vi "DAQX mod 1SDI v02.vi"(0 "resource name":refnum<k15>="PXI1Slot2", 1 "close (T)":bool=TRUE, 2 "Record Data":bool, 3 "numSamples":i32=-1, 4 "max time (s)":dbl=10.0 caption="max time", 5 "min sample rate":dbl=100000000.0, 6 "File location":path, 7 "error in":errorcluster, 8 "reference position":dbl=50.0, 9 "Additional text":string, 10 "Type of measurement":T2, 11 "Name root":string, 13 "channel parameters":T4(array[cluster])=[{"channel name"="0", "input impedance"=0, "maximum input frequency"=30000000.0, "vertical coupling"=1, "probe attenuation"=1.0, "vertical range"=2.0, "vertical offset"=0.0, "channel enabled"=TRUE}, {"channel name"="1", "input impedance"=0, "maximum input frequency"=30000000.0, "vertical coupling"=1, "probe attenuation"=1.0, "vertical range"=2.0, "vertical offset"=0.0, "channel enabled"=TRUE}] {"input impedance" items=["1 mega ohm"=0, "50 ohms"=2]; "vertical coupling" items=["AC", "DC", "Ground"]}, 15 "reset sn":bool) -> (18 "wfm out":waveform(dbl)[](array[waveform]), 22 "Parameters values file":string, 24 "actualSamples 0":i32, 26 "actualSamples 1":i32, 27 "error out":errorcluster caption="error out final")   [LabVIEW 2013]
doc: "Configures and acquires data from an NI-SCOPE high-speed digitizer.\n--------------------\n\nThis Express VI is configured as follows:\n\nDevice: PXI1Slot2 (PXI-5122)\nSample Rate (S/s): 100M\nRecord length: 2k\nAcquisition Mode: N Samples\nChannel 0\n - Range (V): 2\n - Offset (V): 0\n - Probe attenuation: 1\n - Coupling: \n - Input impedence: 1 \n - Bandwidth (Hz): 0\nChannel 1\n - Range (V): 2\n - Offset (V): 0\n - Probe attenuation: 1\n - Coupling: \n - Input impedence: 1 \n - Bandwidth (Hz): 0\nImmediate"
uses:
  <instrlib>/niScope/Controls/niScope vertical coupling.ctl
  Strict Type Defs/type_meas_enum.ctl
  <instrlib>/niScope/Controls/niScope timestamp type.ctl
  <instrlib>/niScope/Acquire/Fetch/niScope Multi Fetch Binary 16.vi
  <instrlib>/niScope/Acquire/Fetch/niScope Multi Fetch WDT.vi
  <instrlib>/niScope/Configure/Trigger/niScope Configure Trigger Immediate.vi
  Global VIs/shotnoise.vi
panel:
  out "Chan 1 params":T1
  out "Chan 0 params":T1
  out "file location into parameter files":path
  out "size(s)":i32
  out "actual sample rate":dbl
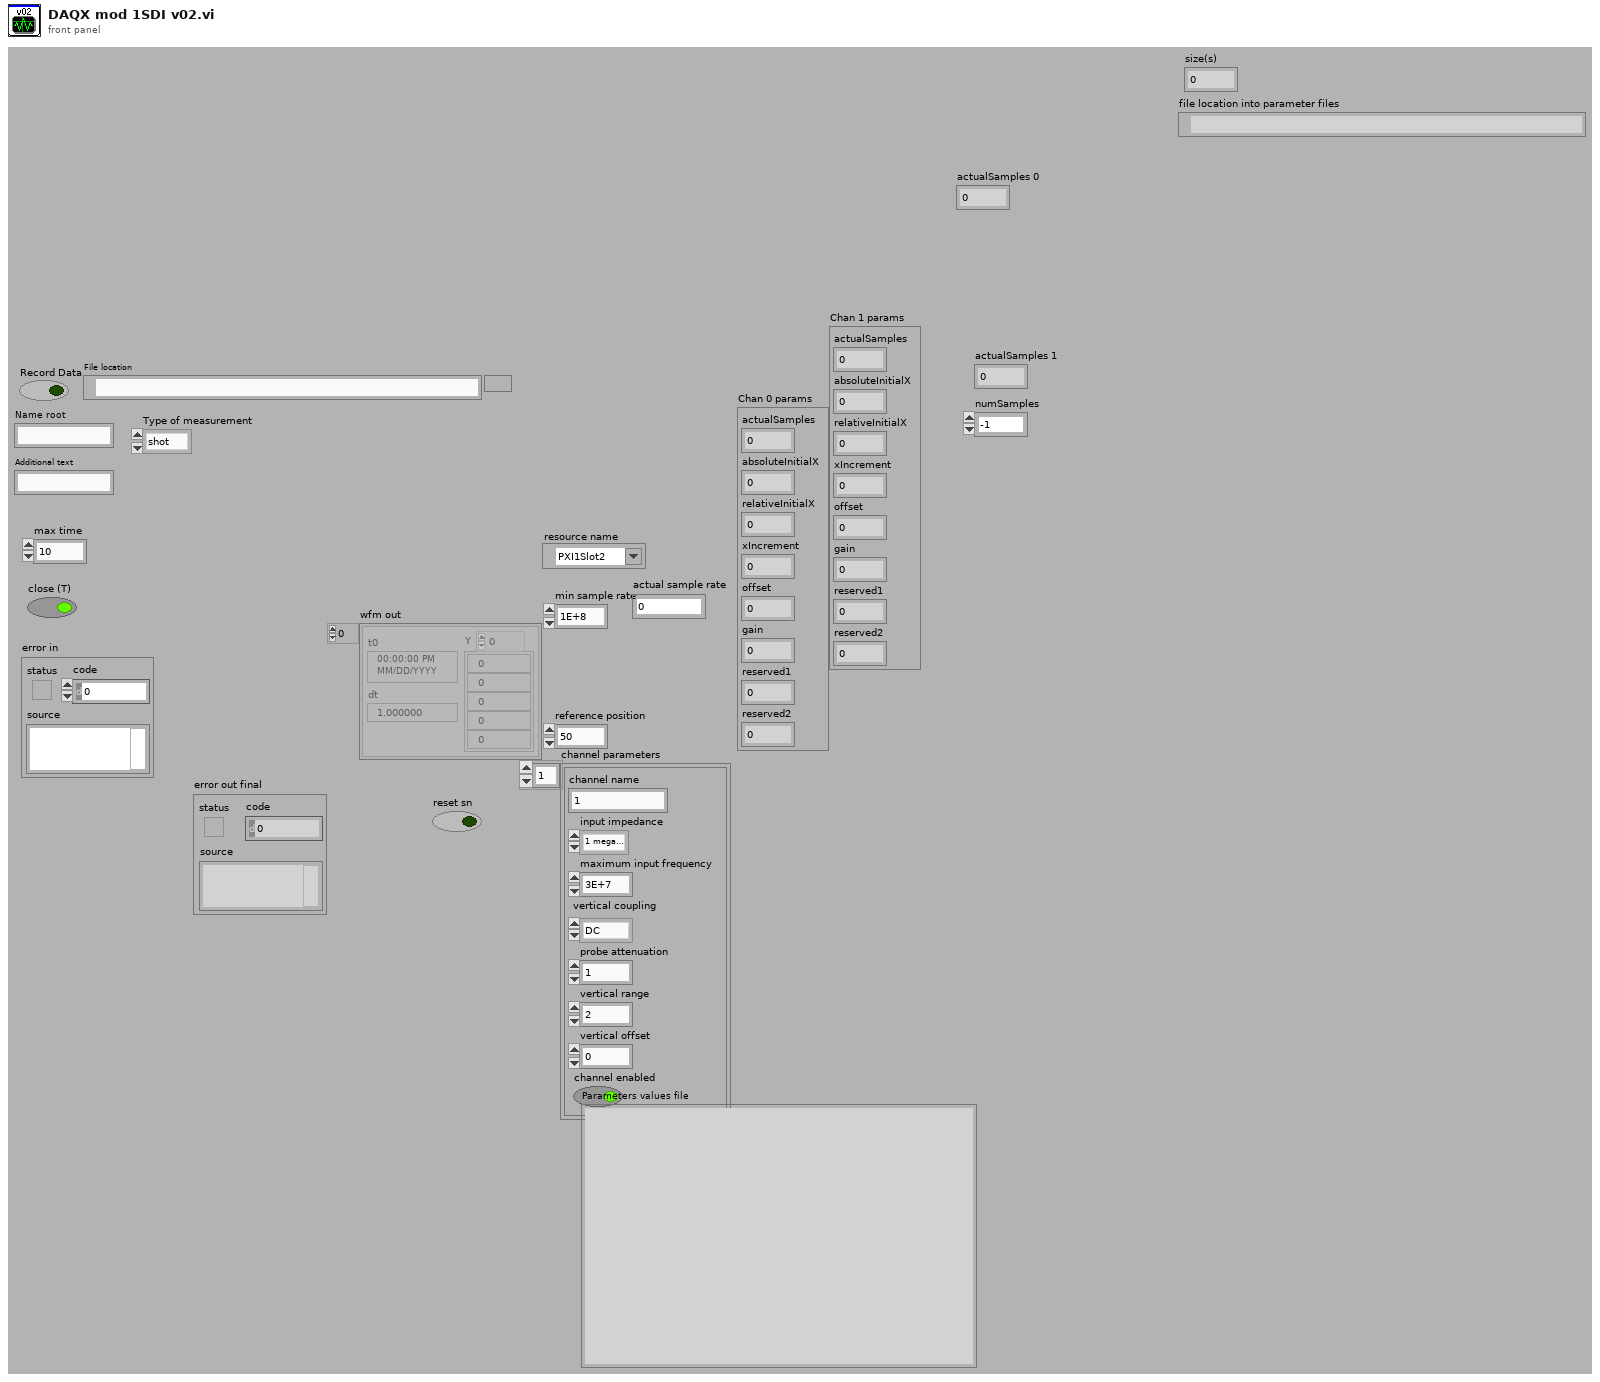
[diagram p1: front panel]
types:
  T1 = cluster{"actualSamples":i32, "absoluteInitialX":dbl, "relativeInitialX":dbl, "xIncrement":dbl, "offset":dbl, "gain":dbl, "reserved1":dbl, "reserved2":dbl}
  T2 = typedef "type_meas_enum.ctl" = enum16{"shot", "x", "p", "electronic"}
  T3 = typedef "niScope vertical coupling.ctl" = i32
  T4 = cluster{"channel name":string, "input impedance":u32, "maximum input frequency":dbl, "vertical coupling":T3, "probe attenuation":dbl, "vertical range":dbl, "vertical offset":dbl, "channel enabled":bool}[]
  T5 = typedef "niScope timestamp type.ctl" = i32
  T6 = cluster{"actualSamples":i32, "absoluteInitialX":dbl, "relativeInitialX":dbl, "xIncrement":dbl, "offset":dbl, "gain":dbl, "reserved1":dbl, "reserved2":dbl}[]
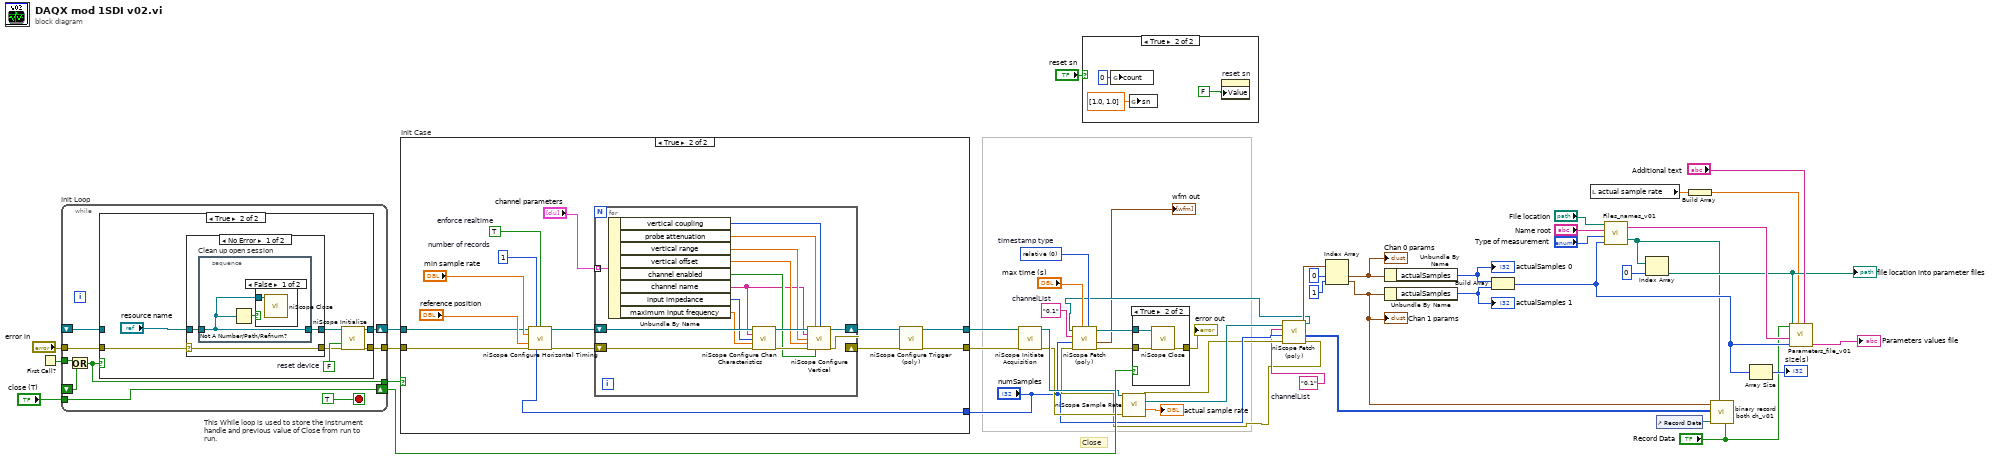
[diagram p0: block diagram]
diagram:
  w11 = "0,1"  # channelList
  w44 = T5 0 items=["relative", "absolute"]  # timestamp type
  w47 = "0,1"  # channelList
  # "This While loop is used to store the instrument handle and previous value of Close from run to run."
  # "Close"
  n1 = First Call?() -> (First Call?: T/F=w43:bool)
  n2 = while "Init Loop" {
    tunnel: w43 -> [w58]
    shift-right: [w57] -> w39
    shift-left: _ -> [w54]
    tunnel: "close (T)" -> [w57]
    shift-right: [w56] -> w42
    shift-left: _ -> [w55]
    tunnel: [w52] -> w41
    tunnel: "error in" -> [w51]
    tunnel: [w50] -> w40
    stop <- TRUE ("stopInit") stop-if-true
    n3 = Or(x=w58, y=w54) -> (x .or. y?=w50:bool)
    n4 = case "Select_Init" shown="True" w50 {
      tunnel: [w60 w65] -> w56
      tunnel: w55 -> [w60 _]
      tunnel: [w59 w64] -> w52
      tunnel: w51 -> [w59 w63]
      frame False {
      }
      frame True {
        w66 = FALSE  # reset device
        n5 = case shown="No Error" w63 {
          selector: w63 -> [w68 w74]
          tunnel: [w70 w75] -> w67
          tunnel: "resource name" -> [w69 w75]
          tunnel: [w68 w74] -> w62
          frame No Error {
            n6 = stacked-sequence "Clean up open session" {
              tunnel: w69 -> [w71]
              tunnel: [w71] -> w70
              frame #0 {
                n7 = Not A Number/Path/Refnum?(number/path/refnum=w71) -> (NaN/Path/Refnum?=w72:bool)
                n8 = case shown="False" w72 {
                  tunnel: w71 -> [w73 _]
                  frame False {
                    n9 = call <instrlib>:"niScope Close.vi"("instrument handle"=w73) -> ()  [unwired: 1 in, 14 out]
                  }
                  frame True {
                  }
                }
              }
            }
          }
          frame Error {
          }
        }
        n10 = call <instrlib>:"niScope Initialize.vi"("resource name"=w67, "reset device"=w66, "error in"=w62) -> ("instrument handle"=w65:refnum<k15>, "error out"=w64:errorcluster)  [unwired: 2 in, 9 out]
      }
    }
  }
  n11 = case "Init Case" shown="True" w40 {
    tunnel: w41 -> [w76 w82]
    tunnel: [w76 w84] -> w46
    tunnel: [w77 w85] -> w45
    tunnel: w42 -> [w77 w83]
    tunnel: "numSamples" -> [_ w78]
    frame False {
    }
    frame True {
      w90 = 1  # number of records
      w91 = TRUE  # enforce realtime
      n12 = call <instrlib>:"niScope Configure Horizontal Timing.vi"("instrument handle"=w83, "number of records"=w90, "enforce realtime"=w91, "min sample rate"="min sample rate", "reference position"="reference position", "error in"=w82, "min record length"=w78) -> ("instrument handle out"=w86:refnum<k15>, "error out"=w87:errorcluster)  [unwired: 7 out]
      n13 = for {
        shift-right: [w94] -> w79
        shift-left: w87 -> [w106]
        shift-right: [w93] -> w80
        shift-left: w86 -> [w105]
        tunnel: "channel parameters" -> [w102] mode=indexing
        n14 = Unbundle By Name(w102) -> ("vertical coupling"=w99:T3, "probe attenuation"=w98:dbl, "vertical range"=w97:dbl, "vertical offset"=w96:dbl, "channel enabled"=w95:bool, "channel name"=w92:string, "input impedance"=w100:u32, "maximum input frequency"=w101:dbl)
        n15 = call <instrlib>:"niScope Configure Chan Characteristics.vi"("instrument handle"=w105, "channels"=w92, "input impedance"=w100, "maximum input frequency"=w101, "error in"=w106) -> ("instrument handle out"=w104:refnum<k15>, "error out"=w103:errorcluster)  [unwired: 9 out]
        n16 = call <instrlib>:"niScope Configure Vertical.vi"("instrument handle"=w104, "probe attenuation"=w98, "vertical coupling"=w99, "channels"=w92, "vertical range"=w97, "vertical offset"=w96, "error in"=w103, "channel enabled"=w95) -> ("instrument handle out"=w93:refnum<k15>, "error out"=w94:errorcluster)  [unwired: 6 out]
      }
      n17 = call-poly <instrlib>:"niScope Configure Trigger (poly).vi"("instrument handle"=w80, "error in"=w79) -> ("instrument handle out"=w85:refnum<k15>, "error out"=w84:errorcluster)  [unwired: 12 out]
    }
  }
  n18 = call <instrlib>:"niScope Initiate Acquisition.vi"("instrument handle"=w45, "error in"=w46) -> ("instrument handle out"=w35:refnum<k15>, "error out"=w34:errorcluster)  [unwired: 12 out]
  n19 = case shown="True" "reset sn" {
    frame False {
    }
    frame True {
      n20 = global write "shotnoise.vi" "count"(i64 0 ("count")) -> ()
      n21 = global write "shotnoise.vi" "sn"(dbl[] [1.0, 1.0] ("sn")) -> ()
      n22 = property on="reset sn" class="Bool (strict)"("Value"=FALSE ("reset sn")) -> ()  [unwired: 2 in, 2 out]
    }
  }
  n23 = call <instrlib>:"niScope Sample Rate.vi"("instrument handle"=w35, "error in"=w34) -> ("instrument handle out"=w30:refnum<k15>, "actual sample rate"=→"actual sample rate":dbl, "error out"=w29:errorcluster)  [unwired: 11 out]
  n24 = call-poly <instrlib>:"niScope Fetch (poly).vi"("error in"=w29, "numSamples"="numSamples", "channels"=w11, "instrument handle"=w30) -> ("error out"=w9:errorcluster, "wfm"=w8:i16[][], "wfm info"=w28:T6, "instrument handle out"=w10:refnum<k15>)  [unwired: 1 in, 3 out]
  n25 = call-poly <instrlib>:"niScope Fetch (poly).vi"("timestamp Type"=w44, "timeout"="max time (s)", "error in"=w9, "numSamples"="numSamples", "channels"=w47, "instrument handle"=w10) -> ("error out"=w6:errorcluster, "wfm"=→"wfm out":waveform(dbl)[], "instrument handle out"=w33:refnum<k15>)  [unwired: 3 out]
  n26 = case shown="True" w39 {
    tunnel: w6 -> [w110 w113]
    tunnel: [w110 w112] -> w49
    tunnel: w33 -> [_ w111]
    frame False {
    }
    frame True {
      n27 = call <instrlib>:"niScope Close.vi"("instrument handle"=w111, "error in"=w113) -> ("error out"=w112:errorcluster)  [unwired: 13 out]
    }
  }
  "error out" <- w49
  n28 = Index Array(array=w28, index #1=0 ("index"), index #2=1 ("index")) -> (element #1=w25:T1, element #2=w2:T1)
  "Chan 0 params" <- w25
  "Chan 1 params" <- w2
  n29 = Unbundle By Name(w25) -> ("actualSamples"=w24:i32)
  "actualSamples 0" <- w24
  n30 = Unbundle By Name(w2) -> ("actualSamples"=w4:i32)
  "actualSamples 1" <- w4
  n31 = Build Array(w24, w4) -> (w13:i32[])
  n32 = local read "actual sample rate"() -> (w15:dbl)
  n33 = call "Files_names_v01.vi"("actualSamples\narray"=w13, "Type of\nmeasurement"="Type of measurement", "Name root"="Name root", "File location"="File location") -> ("Files path array"=w1:path[], "Files name array"=w20:string[])
  n34 = Index Array(array=w1, index=0) -> (element=w17:path)
  "file location into parameter files" <- w17
  n35 = control-ref of="Record Data"() -> (w3:refnum<vi>)
  n36 = Build Array(w15) -> (w14:dbl[])
  n37 = call "binary record both ch_v01.vi"("Record"="Record Data", "Files path array"=w1, "reference"=w3, "wfm"=w8, "Chan 1 params"=w2) -> ()  [unwired: 7 in]
  n38 = Array Size(array=w13) -> (size(s)=→"size(s)":i32)
  n39 = call "Parameters_file_v01.vi"("Additional text"="Additional text", "actual sample rate array"=w14, "actualSamples array"=w13, "Files name array"=w20, "File location"=w17, "Record"="Record Data") -> ("Full text"=→"Parameters values file":string)  [unwired: 3 in]
